vi "Trigger Delay.vi"(8 "input valid":bool=TRUE, 10 "Count to skip":u32) -> (0 "output valid":bool)   [LabVIEW 2018]
uses:
  <instrlib>/_niInstr/Basic Elements/v1/FPGA/Private/Count Down U32.vi
  <instrlib>/_niInstr/Basic Elements/v1/FPGA/niInstr Basic Elements v1 FPGA.lvlib
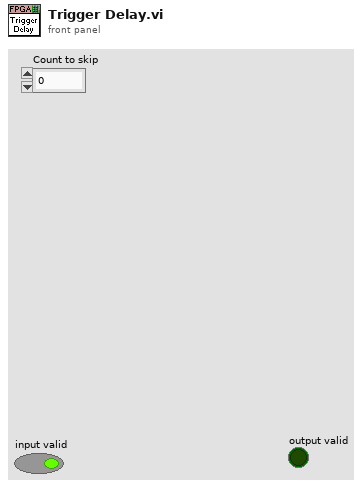
[diagram p1: front panel]
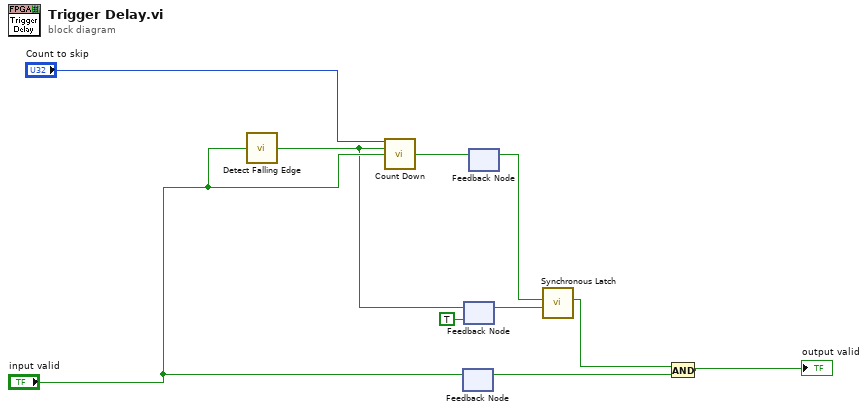
[diagram p0: block diagram]
diagram:
  n1 = call <instrlib>:"Detect Falling Edge.vi"("signal"="input valid") -> ("edge detected"=w2:bool)  [unwired: 14 in]
  n2 = call-poly <instrlib>:"Count Down.vi"("count in"="Count to skip", "load"=w2, "decrement"="input valid") -> ("terminal count"=w9:bool)  [unwired: 11 in, 1 out]
  n3 = feedback #1() -> (w7:bool)  [unwired: 1 in]
  n4 = feedback-in #1("input valid") -> ()
  n5 = feedback #2(TRUE) -> (w8:bool)
  n6 = feedback-in #2(w2) -> ()
  n7 = feedback #3() -> (w3:bool)  [unwired: 1 in]
  n8 = feedback-in #3(w9) -> ()
  n9 = call <instrlib>:"Synchronous Latch.vi"("clear"=w8, "set"=w3) -> ("out"=w5:bool)  [unwired: 9 in]
  n10 = And(x=w5, y=w7) -> (x .and. y?=→"output valid":bool)
